vi "Rinocloud_HTTP_append.vi"(5 "chunk":string, 8 "id":string) -> (0 "error out":errorcluster, 2 "body":string, 3 "headers":string)   [LabVIEW 2013]
uses:
  Rinocloud_global_variable.vi
  <vilib>/httpClient/POSTBuffer.vi
  <vilib>/httpClient/LabVIEWHTTPClient.lvlib
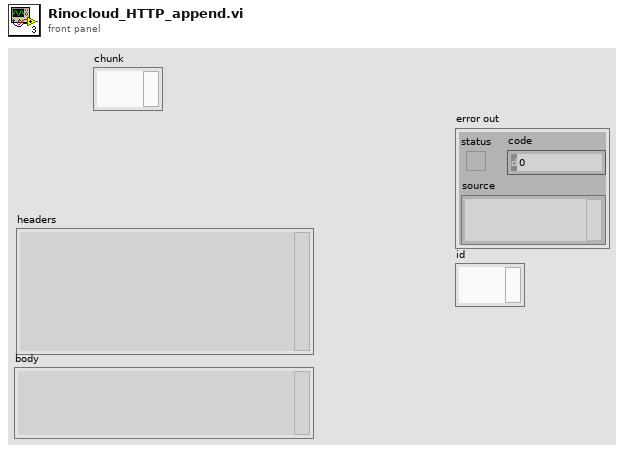
[diagram p1: front panel]
types:
  T1 = typedef "LabVIEWHTTPClient.lvlib/ClientHandle.ctl" = refnum<k1>
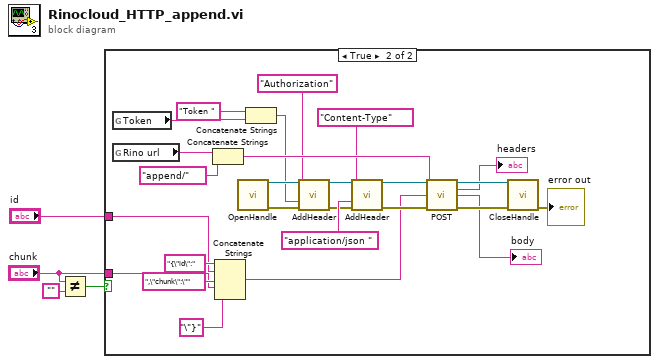
[diagram p0: block diagram]
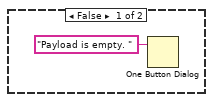
[diagram p2: hidden frame]
diagram:
  n1 = Not Equal?(x="chunk", y="") -> (x != y?=w1:bool)
  n2 = case shown="True" w1 {
    tunnel: "id" -> [_ w7]
    tunnel: "chunk" -> [_ w6]
    frame False {
      n3 = One Button Dialog(message="Payload is empty. ") -> ()  [unwired: 1 in, 1 out]
    }
    frame True {
      n4 = global read "Rinocloud_global_variable.vi" "Token"() -> (w23:string)
      n5 = global read "Rinocloud_global_variable.vi" "Rino url"() -> (w29:string)
      n6 = Concatenate Strings(w29, "append/" ("Combo Box 2")) -> (w31:string)
      n7 = Concatenate Strings("{\"id\":" ("string"), w7, ",\"chunk\":\"" ("string"), w6, "\"}" ("string")) -> (w10:string)
      n8 = call <vilib>:"OpenHandle.vi"() -> ("client handle out"=w27:T1, "error out"=w24:errorcluster)  [unwired: 14 in]
      n9 = Concatenate Strings("Token " ("value"), w23) -> (w25:string)
      n10 = call <vilib>:"AddHeader.vi"("client handle"=w27, "header"="Authorization" ("url"), "value"=w25, "error in (no error)"=w24) -> ("client handle out"=w16:T1, "error out"=w14:errorcluster)  [unwired: 10 in]
      n11 = call <vilib>:"AddHeader.vi"("client handle"=w16, "header"="Content-Type", "value"="application/json ", "error in (no error)"=w14) -> ("client handle out"=w15:T1, "error out"=w13:errorcluster)  [unwired: 10 in]
      n12 = call-poly <vilib>:"POST.vi"("client handle"=w15, "url"=w31, "buffer"=w10, "error in (no error)"=w13) -> ("client handle out"=w22:T1, "headers"=→"headers":string, "body"=→"body":string, "error out"=w21:errorcluster)  [unwired: 8 in]
      n13 = call <vilib>:"CloseHandle.vi"("client handle"=w22, "error in (no error)"=w21) -> ("error out"=→"error out":errorcluster)  [unwired: 13 in]
    }
  }
